vi "Fetch Multiple Measurements.vi"   [LabVIEW 2020, in "Agilent 681x Series.lvlib"]
doc: "Fetches current or voltage data.\n\n<B>Note:</B>\n\nUse this VI only with other low-level VIs. The high-level VIs automatically incorporate this functionality. This VI does not check the instrument status. If you want to check the instrument status, call the Error Query VI at the conclusion of the sequence."
uses:
  <instrlib>/Agilent 681x Series/Agilent 681x Series.lvlib
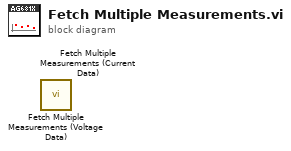
[diagram p0: block diagram]
diagram:
  n1 = call <instrlib>:"Fetch Multiple Measurements (Voltage Data).vi"() -> ()  [unwired: 11 in, 5 out]
  n2 = call <instrlib>:"Fetch Multiple Measurements (Current Data).vi"() -> ()  [unwired: 11 in, 5 out]
